vi "Clear Phase Accumulation.vi"(8 "error in (no error)":errorcluster, 10 "Modulation Format (1: Dual Modulation)":u16(ring)=1 items=["Custom"=0, "Dual Modulation"=1, "Dual ARB"=2, "Multitone"=3, "Two-tone"=6], 11 "VISA resource name":refnum<visa-resource-name>) -> (0 "error out":errorcluster, 3 "VISA resource name out":refnum<visa-resource-name>)   [LabVIEW 2014, in "Agilent PSG MXG Series.lvlib"]
doc: "Clears the phase accumulation and so zero phase shift.\nWhen the Baseband Frequency Offset is non-zero, the hardware rotator accumulates phase-shift of the baseband signal. This residual phase remains even after the offset value is returned to zero.\nWhile there is a non-zero residual phase present in the signal, the DAC Over-Range Protection feature will automatically prevent DAC overrange errors from occurring by scaling the signal down by 1/square root of 2.\n\n<B>Notes:</B>\n(1) This VI is valid only in N5162A, N5182A, N5172B, N5182B.\n\n(2) For N5162A, N5182A, this VI is valid only when the instrument installs <B>Option 651</B> or <B>Option 652</B> or <B>Option 654</B> (Internal baseband generator).\n\n(3) For N5172B, N5182B, this VI is valid only when the instrument installs <B>Option 431</B>."
uses:
  Agilent PSG MXG Series.lvlib
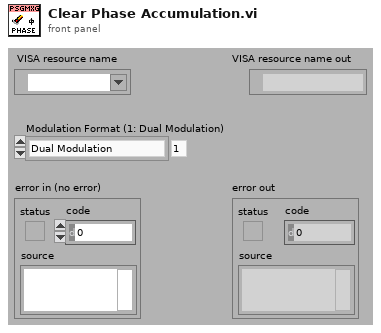
[diagram p1: front panel]
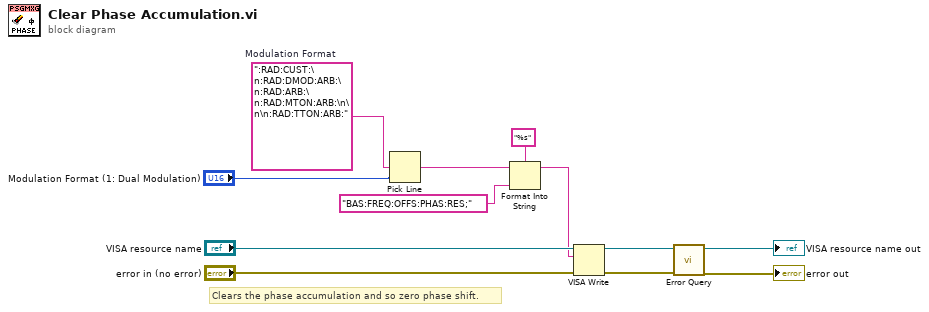
[diagram p0: block diagram]
diagram:
  w5 = ":RAD:CUST:\n:RAD:DMOD:ARB:\n:RAD:ARB:\n:RAD:MTON:ARB:\n\n\n:RAD:TTON:ARB:"  # Modulation Format
  # "Clears the phase accumulation and so zero phase shift."
  n1 = Pick Line(multi-line string=w5, line index="Modulation Format (1: Dual Modulation)") -> (output string=w2:string)  [unwired: 1 out]
  n2 = Format Into String(format string="%s", initial string=w2, "BAS:FREQ:OFFS:PHAS:RES;") -> (resulting string=w3:string)  [unwired: 1 in, 1 out]
  n3 = VISA Write(VISA resource name="VISA resource name", write buffer=w3, error in (no error)="error in (no error)") -> (VISA resource name out=w10:refnum<visa-resource-name>, error out=w9:errorcluster)  [unwired: 1 out]
  n4 = call "Error Query.vi"("error in (no error)"=w9, "VISA resource name"=w10) -> ("error out"=→"error out":errorcluster, "VISA resource name out"=→"VISA resource name out":refnum<visa-resource-name>)  [unwired: 8 out]
